vi "Channel Count.vi"(8 "error in (no error)":errorcluster, 11 "Framework Configuration in":refnum<class "Framework Configuration.lvclass">) -> (0 "error out":errorcluster, 2 "channel count":i32, 3 "Framework Configuration out":refnum<class "Framework Configuration.lvclass">)   [LabVIEW 2021, in "DSF Core.lvlib" / "Framework Configuration.lvclass"]
uses:
  Framework Configuration.lvclass
  Framework Configuration.lvclass/Framework Configuration.ctl
  Plugin/Plugin Configuration.lvclass
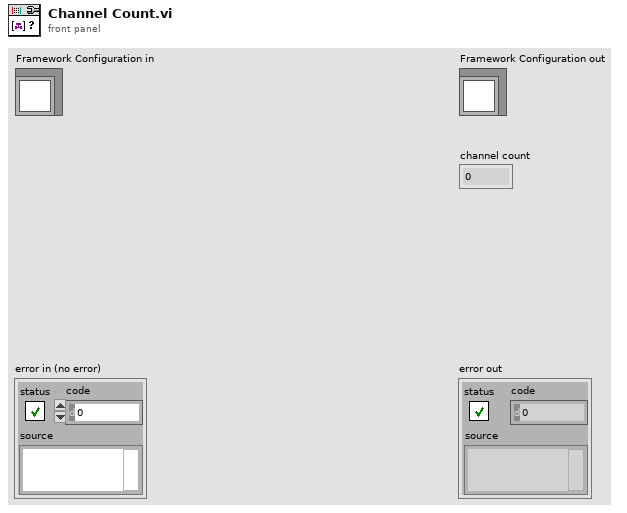
[diagram p1: front panel]
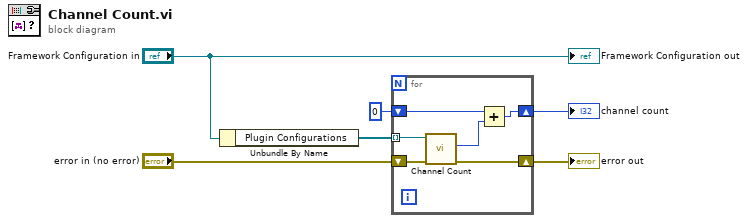
[diagram p0: block diagram]
diagram:
  n1 = Unbundle By Name("Framework Configuration in") -> ("Plugin Configurations"=w5:refnum<class "Plugin Configuration.lvclass">[])
  n2 = for {
    shift-right: [w11] -> w3
    shift-left: "error in (no error)" -> [w12]
    tunnel: w5 -> [w10] mode=indexing
    shift-right: [w7] -> w4
    shift-left: 0 ("channel count") -> [w9]
    n3 = call-dynamic "Channel Count.vi"("error in (no error)"=w12, "Plugin Configuration in"=w10) -> ("error out"=w11:errorcluster, "channel count"=w8:i32)  [unwired: 7 in, 1 out]
    n4 = Add(x=w9, y=w8) -> (x+y=w7:i32)
  }
  "error out" <- w3
  "channel count" <- w4
  "Framework Configuration out" <- "Framework Configuration in"
